vi "test - Response of CSM Send Message.vi"(8 "error in (no error)":errorcluster, 11 "TestCase in":refnum<class "testcase-Basic-Function.lvclass">) -> (0 "error out":errorcluster, 3 "TestCase out":refnum<class "testcase-Basic-Function.lvclass">)   [LabVIEW 2017, in "testcase-Basic-Function.lvclass"]
uses:
  testcase-Basic-Function.lvclass
  src/user.lib/_NEVSTOP/Communicable State Machine(CSM)/AdvanceAPI/CSM - Revert Arguments-Safe String.vi
  src/user.lib/_NEVSTOP/Communicable State Machine(CSM)/_Shared/Trim Single-line Text.vi
  src/user.lib/_NEVSTOP/Communicable State Machine(CSM)/AdvanceAPI/CSM - Make String Arguments Safe.vi
  src/user.lib/_NEVSTOP/Communicable State Machine(CSM)/AdvanceAPI/CSM - Break Down Multiple States String.vi
  src/user.lib/_NEVSTOP/Communicable State Machine(CSM)/AdvanceAPI/CSM - Compact Multiple States.vi
  src/user.lib/_NEVSTOP/Communicable State Machine(CSM)/AdvanceAPI/CSM - Keywords.vi
  src/user.lib/_NEVSTOP/Communicable State Machine(CSM)/Communicable State Machine.lvlib
  <vilib>/addons/_JKI Toolkits/VI Tester/TestCase.llb/TestCase.lvclass
  C:/Program Files (x86)/National Instruments/LabVIEW 2017/vi.lib/addons/_JKI Toolkits/VI Tester/TestCase.llb/TestCase.lvclass
panel:
  in  "response not empty in error handler":bool
  out "State History":string
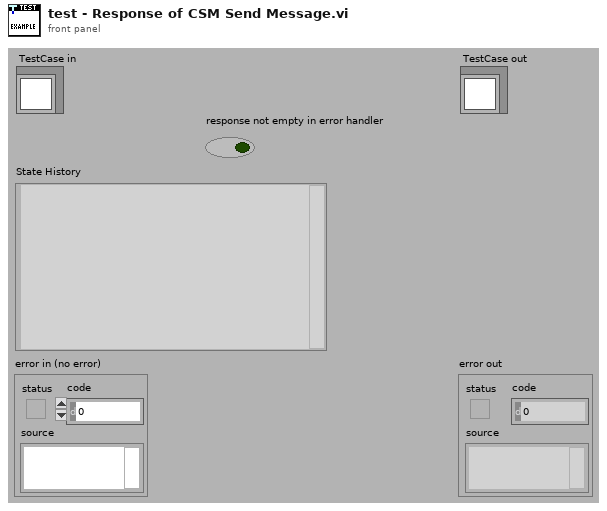
[diagram p1: front panel]
types:
  T1 = enum32{"Invalid", "Standard", "Closed", "Hidden", "Minimized", "Maximized"}
  T2 = enum32{"invalid app kind", "Development System", "Run Time System", "Student Edition", "Embedded LabVIEW", "Evaluation", "Custom"}
  T3 = typedef "Communicable State Machine.lvlib/_CSM_Response Source Message.ctl" = cluster{"‘State":string, "’Arguments":string, "’Error":errorcluster}
  T4 = cluster{"Current VI Reference":refnum<vi>, "Close Panel on Exit?":bool}
  T5 = cluster{"Core":cluster{"Current VI Reference":refnum<vi>, "Close Panel on Exit?":bool}, "Your Boolean data":bool, "Your string data":string}
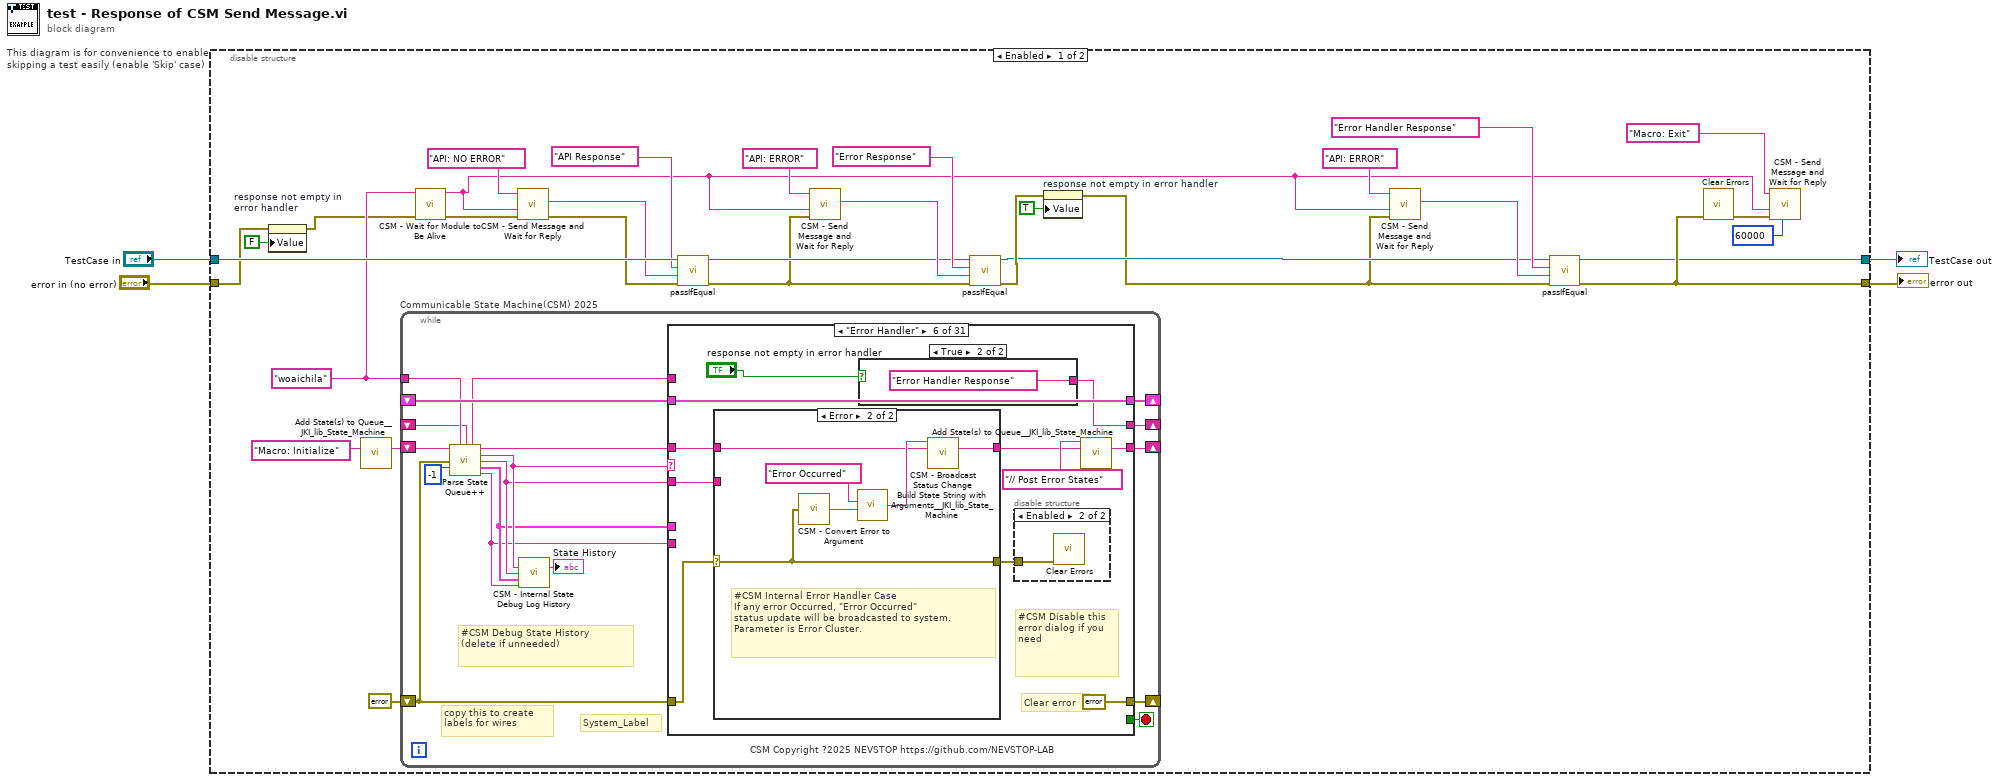
[diagram p0: block diagram]
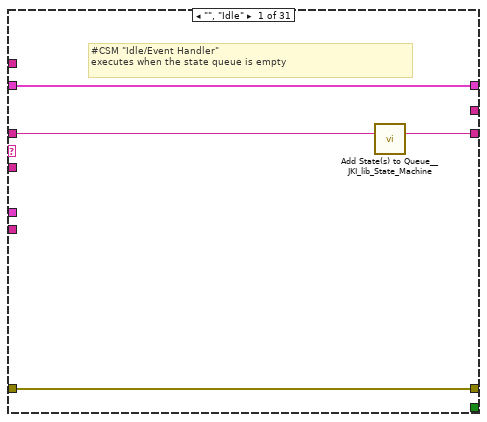
[diagram p2: hidden frame]
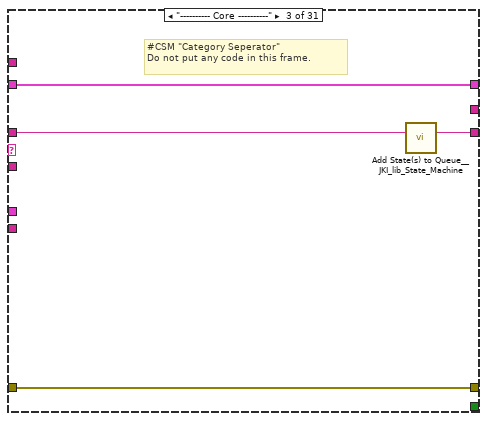
[diagram p4: hidden frame]
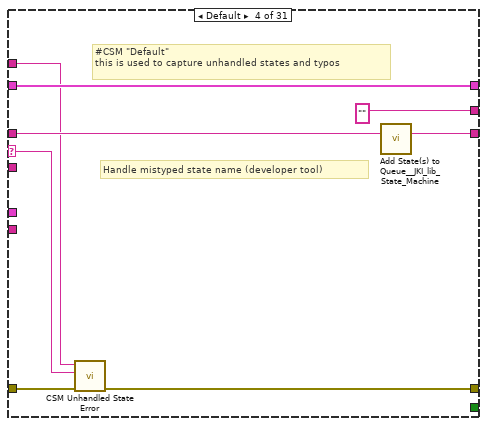
[diagram p5: hidden frame]
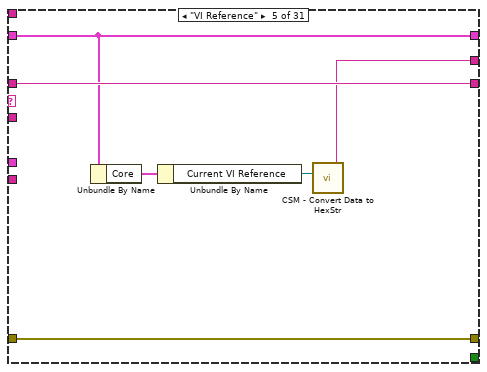
[diagram p6: hidden frame]
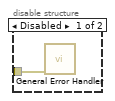
[diagram p8: hidden frame]
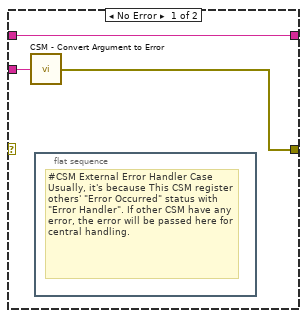
[diagram p9: hidden frame]
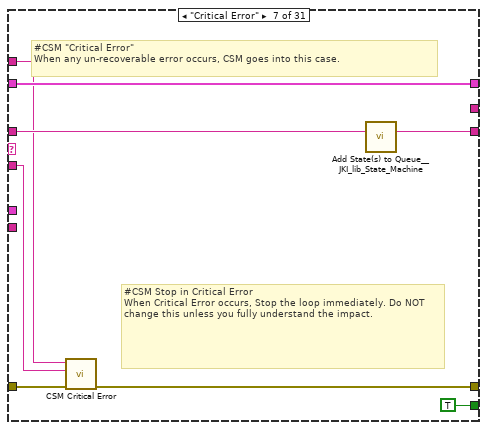
[diagram p10: hidden frame]
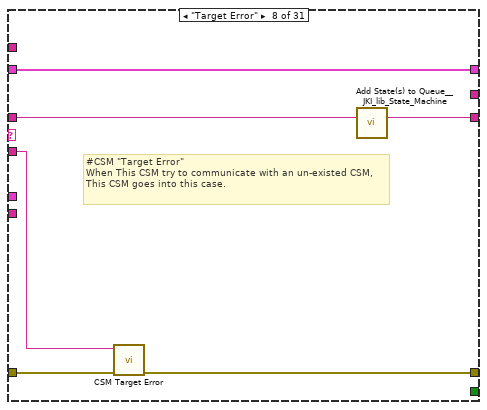
[diagram p11: hidden frame]
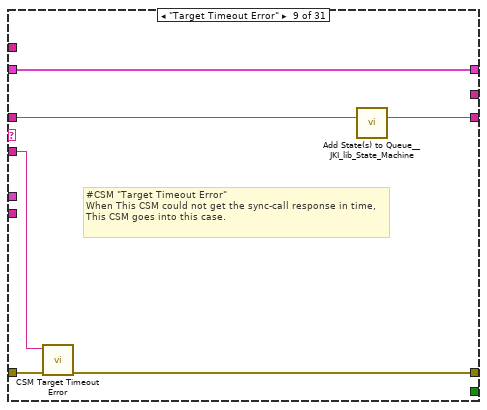
[diagram p12: hidden frame]
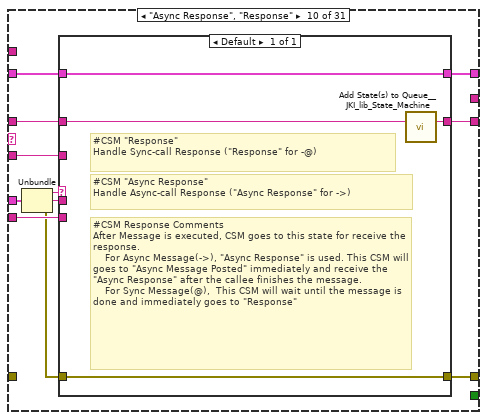
[diagram p13: hidden frame]
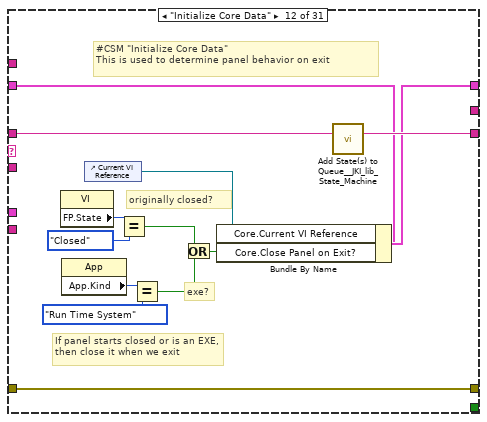
[diagram p15: hidden frame]
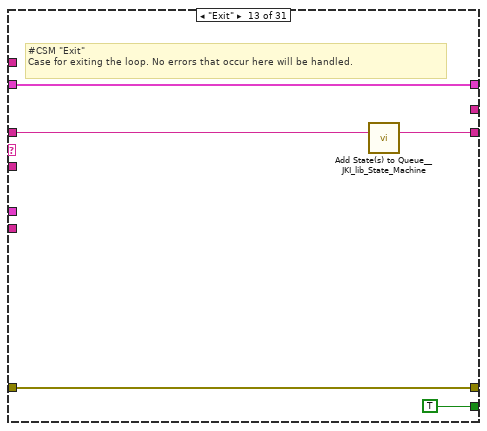
[diagram p16: hidden frame]
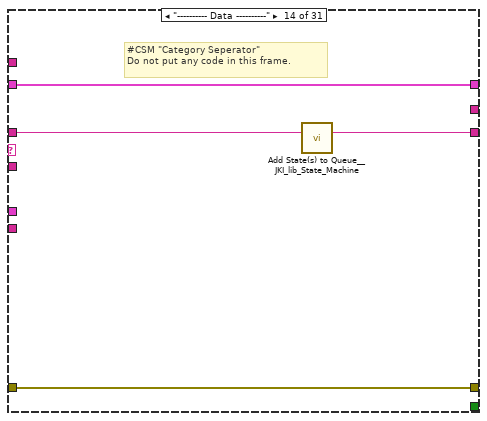
[diagram p17: hidden frame]
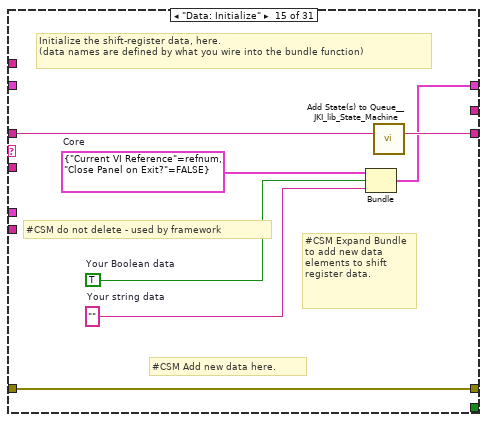
[diagram p18: hidden frame]
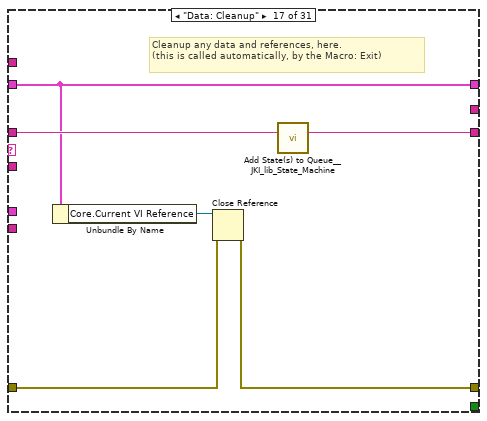
[diagram p20: hidden frame]
diagram:
  n1 = disable-structure "This diagram is for convenience to enable skipping a test easily (enable 'Skip' case)" shown="Enabled" {
    disable-tunnel: "TestCase in" -> [w35 w321]
    disable-tunnel: [w6 w319] -> w1
    disable-tunnel: [w8 w320] -> w3
    disable-tunnel: "error in (no error)" -> [w17 w318]
    frame Enabled {
      w30 = "woaichila" ("Name (\"\" to Use UUID)")
      n2 = property on="response not empty in error handler" class="Bool (strict)"(error in=w17, "Value"=FALSE ("response not empty in error handler")) -> (error out=w16:errorcluster)  [unwired: 1 in, 1 out]
      n3 = call <vilib>:"Add State(s) to Queue__JKI_lib_State_Machine.vi"("State(s) in (\"\")"="Macro: Initialize" ("Init State(\"Macro: Initialize\")")) -> ("States Out"=w32:string)  [unwired: 14 in]
      n4 = while "Communicable State Machine(CSM) 2025" {
        shift-right: [w48] -> _
        shift-left: _ -> [w47]
        shift-right: [w51] -> _
        shift-left: errorcluster {"status"=FALSE, "code"=0, "source"=""} ("error out") -> [w46]
        shift-right: [w50] -> _
        shift-left: w32 -> [w52]
        tunnel: w30 -> [w44]
        shift-right: [w45] -> _
        shift-left: _ -> [w38]
        stop <- w49 stop-if-true
        # "#CSM Debug State History\n(delete if unneeded)"
        # "copy this to create labels for wires"
        # "System_Label"
        # "CSM Copyright ?2025 NEVSTOP https://github.com/NEVSTOP-LAB"
        n5 = call "Parse State Queue++.vi"("State Queue"=w52, "Name (\"\" to Use UUID)"=w44, "Response Arguments"=w38, "Previous Error"=w46, "Dequeue (1 ms)"=-1 ("Timeout")) -> ("Name Used"=w39:string, "Remaining States"=w53:string, "Current State"=w43:string, "Arguments"=w42:string, "Additional Information"=w41:T3, "Source CSM"=w40:string)  [unwired: 5 in]
        n6 = call "CSM - Internal State Debug Log History.vi"("State"=w43, "Arguments (\"\")"=w42, ">> Response Source Message >>"=w41, "Source (\"\")"=w40) -> ("Debug Log"=→"State History":string)  [unwired: 11 in]
        n7 = case shown="\"Error Handler\"" w43 {
          selector: w43 -> [_ _ _ w67 _ _ _ _ _ _ _ _ _ _ _ _ _ _ _ _ _ _ _ _ _ _ _ _ _ _ _]
          tunnel: w53 -> [w54 w59 w64 w71 w77 w85 w107 w113 w119 w127 w138 w152 w157 w161 w168 w170 w177 w181 w185 w191 w206 w275 w280 w287 w289 w293 w298 w302 w309 w313 w317]
          tunnel: w42 -> [_ _ _ _ _ w84 w103 w112 w117 w126 _ _ _ _ _ _ _ _ _ w186 w200 _ _ _ _ _ _ w300 _ _ _]
          tunnel: w47 -> [w55 w58 w61 w69 w76 w88 w108 w114 w120 w129 w137 w145 w155 w158 _ w169 w172 w178 w183 w189 w202 w272 w277 w284 w288 w292 w297 w301 w306 w310 w314]
          tunnel: [w56 w60 w62 w65 w78 errorcluster {"status"=FALSE, "code"=0, "source"=""} ("error out") w104 w110 w116 w132 w139 w149 w154 w159 w165 w171 w173 w179 w182 w187 w203 w273 w278 w285 w290 w294 errorcluster {"status"=TRUE, "code"=-1, "source"="xxxx"} ("error out") w303 w307 w311 w315] -> w51
          tunnel: w46 -> [w56 w60 w62 w72 w78 w86 w109 w111 w118 _ w139 w149 w154 w159 w165 w171 w174 w179 w182 w188 w204 w273 w278 w285 w290 w294 _ w303 w307 w311 w315]
          tunnel: [w57 w59 w63 w70 w77 w81 w106 w115 w121 w128 w138 w151 w156 w160 w167 w170 w176 w180 w184 w190 w205 w274 w279 w286 w289 w293 w298 w302 w308 w312 w316] -> w50
          tunnel: [_ _ _ _ _ _ TRUE _ _ _ _ _ TRUE _ _ _ _ _ _ _ _ _ _ _ _ _ _ _ _ _ _] -> w49
          tunnel: [w55 w58 w61 w69 w76 w88 w108 w114 w120 w130 w137 w150 w155 w158 w166 w169 w172 w178 w183 w189 w202 w272 w277 w284 w288 w292 w297 w301 w306 w310 w314] -> w48
          tunnel: w40 -> [_ _ _ _ _ _ _ _ _ w124 _ _ _ _ _ _ _ _ _ _ _ _ _ _ _ _ _ _ _ _ _]
          tunnel: w41 -> [_ _ _ _ _ _ _ _ _ w131 _ _ _ _ _ _ _ _ _ _ _ _ _ _ _ _ _ _ _ _ _]
          tunnel: [_ _ _ "" w73 w80 _ _ _ _ _ _ _ _ _ _ _ _ _ _ _ _ _ _ _ "API Response" "Error Response" w299 _ _ _] -> w45
          tunnel: w39 -> [_ _ _ w66 _ _ w102 _ _ _ _ _ _ _ _ _ _ _ _ _ _ _ _ _ _ _ _ _ _ _ _]
          frame "", "Idle" {
            # "#CSM \"Idle/Event Handler\"\nexecutes when the state queue is empty"
            n8 = call <vilib>:"Add State(s) to Queue__JKI_lib_State_Machine.vi"("State(s) in (\"\")"=w54) -> ("States Out"=w57:string)  [unwired: 14 in]
          }
          frame "CSM Documentation" {
            # "#CSM README FIRST\n\nCommunicable State Machine(CSM) is a LabVIEW application framework that builds upon JKI State Machine(JKISM). It follows the pattern of JKISM and extends the keywords to describe message communication between modules, including concepts such as Sync-Message, Async-Message, Subscription/Unsubscription of status - essential elements for creating reusable code modules. For more information, please visit the CSM wiki: https://nevstop-lab.github.io/CSM-Wiki/\n\nFor instructions on JKI State Machine, visit: http://jki.net/state-machine/\nFor information about CSM, visit: https://github.com/NEVSTOP-LAB"
            # "#CSM \"Documentation\"\nCase for holding CSM Documenation"
          }
          frame "---------- Core ----------" {
            # "#CSM \"Category Seperator\"\nDo not put any code in this frame."
            n9 = call <vilib>:"Add State(s) to Queue__JKI_lib_State_Machine.vi"("State(s) in (\"\")"=w64) -> ("States Out"=w63:string)  [unwired: 14 in]
          }
          frame Default {
            # "#CSM \"Default\"\nthis is used to capture unhandled states and typos"
            # "Handle mistyped state name (developer tool)"
            n10 = call "CSM Unhandled State Error.vi"("error in (no error)"=w72, "Undefined State"=w67, "CSM Name"=w66) -> ("error out"=w65:errorcluster)  [unwired: 8 in]
            n11 = call <vilib>:"Add State(s) to Queue__JKI_lib_State_Machine.vi"("State(s) in (\"\")"=w71) -> ("States Out"=w70:string)  [unwired: 14 in]
          }
          frame "VI Reference" {
            n12 = Unbundle By Name(w76) -> ("Core"=w75:T4)
            n13 = Unbundle By Name(w75) -> ("Current VI Reference"=w74:refnum<vi>)
            n14 = call "CSM - Convert Data to HexStr.vi"("Variant"=w74) -> ("HEX String (0-9,A-F)"=w73:string)  [unwired: 8 in]
          }
          frame "Error Handler" {
            # "#CSM Disable this error dialog if you need"
            # "Clear error"
            n15 = case shown="Error" w86 {
              selector: w86 -> [_ w96]
              tunnel: [w95 w98] -> w82
              tunnel: w85 -> [w95 w97]
              tunnel: w84 -> [w94 _]
              tunnel: [w93 w96] -> w87
              frame No Error {
                n16 = call "CSM - Convert Argument to Error.vi"("Argument"=w94) -> ("Error"=w93:errorcluster)  [unwired: 4 in]
                n17 = flat-sequence {
                  frame #0 {
                    # "#CSM External Error Handler Case\nUsually, it's because This CSM register others' \"Error Occurred\" status with \"Error Handler\". If other CSM have any error, the error will be passed here for central handling."
                  }
                }
              }
              frame Error {
                # "#CSM Internal Error Handler Case \nIf any error Occurred, \"Error Occurred\" \nstatus update will be broadcasted to system.\nParameter is Error Cluster."
                n18 = call "CSM - Convert Error to Argument.vi"("Error"=w96) -> ("Argument"=w100:string)  [unwired: 4 in]
                n19 = call <vilib>:"Build State String with Arguments__JKI_lib_State_Machine.vi"("Arguments (\"\")"=w100, "State"="Error Occurred" ("Status with Arguments")) -> ("State with Arguments"=w99:string)  [unwired: 4 in]
                n20 = call "CSM - Broadcast Status Change.vi"("Status With Arguments"=w99, "State Queue"=w97) -> ("Remaining States"=w98:string)  [unwired: 13 in]
              }
            }
            n21 = case shown="True" "response not empty in error handler" {
              tunnel: [_ "Error Handler Response"] -> w80
              frame False {
              }
              frame True {
              }
            }
            n22 = disable-structure shown="Enabled" {
              disable-tunnel: w87 -> [w91 w92]
              frame Disabled {
                n23 = call <vilib>:"General Error Handler.vi"("error in (no error)"=w91) -> ()  [unwired: 10 in, 5 out]
              }
              frame Enabled {
                n24 = call <vilib>:"Clear Errors.vi"("error in (no error)"=w92) -> ()  [unwired: 5 in, 2 out]
              }
            }
            n25 = call <vilib>:"Add State(s) to Queue__JKI_lib_State_Machine.vi"("State(s) in Front (\"\")"="// Post Error States", "State(s) in (\"\")"=w82) -> ("States Out"=w81:string)  [unwired: 13 in]
          }
          frame "Critical Error" {
            # "#CSM Stop in Critical Error\nWhen Critical Error occurs, Stop the loop immediately. Do NOT change this unless you fully understand the impact."
            # "#CSM \"Critical Error\"\nWhen any un-recoverable error occurs, CSM goes into this case."
            n26 = call "CSM Critical Error.vi"("error in (no error)"=w109, "Arugments (As Reason)"=w103, "CSM Name"=w102) -> ("error out"=w104:errorcluster)  [unwired: 8 in]
            n27 = call <vilib>:"Add State(s) to Queue__JKI_lib_State_Machine.vi"("State(s) in (\"\")"=w107) -> ("States Out"=w106:string)  [unwired: 14 in]
          }
          frame "Target Error" {
            # "#CSM \"Target Error\"\nWhen This CSM try to communicate with an un-existed CSM, This CSM goes into this case."
            n28 = call "CSM Target Error.vi"("error in (no error)"=w111, "Arguments (As CSM Name)"=w112) -> ("error out"=w110:errorcluster)  [unwired: 9 in]
            n29 = call <vilib>:"Add State(s) to Queue__JKI_lib_State_Machine.vi"("State(s) in (\"\")"=w113) -> ("States Out"=w115:string)  [unwired: 14 in]
          }
          frame "Target Timeout Error" {
            # "#CSM \"Target Timeout Error\"\nWhen This CSM could not get the sync-call response in time, This CSM goes into this case."
            n30 = call "CSM Target Timeout Error.vi"("error in (no error)"=w118, "Arguments (As CSM Name)"=w117) -> ("error out"=w116:errorcluster)  [unwired: 9 in]
            n31 = call <vilib>:"Add State(s) to Queue__JKI_lib_State_Machine.vi"("State(s) in (\"\")"=w119) -> ("States Out"=w121:string)  [unwired: 14 in]
          }
          frame "Async Response", "Response" {
            n32 = Unbundle(w131) -> ("‘State"=w125:string, "’Arguments"=w123:string, "’Error"=w122:errorcluster)
            n33 = case shown="Default" w125 {
              tunnel: [w136] -> w132
              tunnel: w122 -> [w136]
              tunnel: [w135] -> w130
              tunnel: w129 -> [w135]
              tunnel: [w133] -> w128
              tunnel: w127 -> [w134]
              tunnel: w126 -> [_]
              tunnel: w124 -> [_]
              tunnel: w123 -> [_]
              frame Default {
                # "#CSM Response Comments\nAfter Message is executed, CSM goes to this state for receive the response.\n    For Async Message(->), \"Async Response\" is used. This CSM will goes to \"Async Message Posted\" immediately and receive the \"Async Response\" after the callee finishes the message.\n    For Sync Message(@),  This CSM will wait until the message is done and immediately goes to \"Response\""
                # "#CSM \"Async Response\"\nHandle Async-call Response (\"Async Response\" for ->)"
                # "#CSM \"Response\"\nHandle Sync-call Response (\"Response\" for -@)"
                n34 = call <vilib>:"Add State(s) to Queue__JKI_lib_State_Machine.vi"("State(s) in (\"\")"=w134) -> ("States Out"=w133:string)  [unwired: 14 in]
              }
            }
          }
          frame "Async Message Posted" {
            # "#CSM \"Async Message Posted\"\nAfter Async Message is posted (-> or ->| ), CSM goes to this state for post-action.\nYou can use Argument - State to tell which Async Message is called."
          }
          frame "Initialize Core Data" {
            # "#CSM \"Initialize Core Data\"\nThis is used to determine panel behavior on exit"
            # "originally closed?"
            # "exe?"
            # "If panel starts closed or is an EXE, then close it when we exit"
            n35 = property class="VI"() -> ("FP.State"=w142:T1)  [unwired: 2 in, 2 out]
            n36 = property class="App"() -> ("App.Kind"=w148:T2)  [unwired: 2 in, 2 out]
            n37 = control-ref of="Current VI Reference"() -> (w143:refnum<vi>)
            n38 = Equal?(x=w142, y=T1."Closed" ("Front Panel Window:State")) -> (x = y?=w140:bool)
            n39 = Equal?(x=w148, y=T2."Run Time System" ("Application:Kind")) -> (x = y?=w146:bool)
            n40 = Or(x=w140, y=w146) -> (x .or. y?=w144:bool)
            n41 = Bundle By Name(cluster=w145, "Core.Current VI Reference"=w143, "Core.Close Panel on Exit?"=w144) -> (w150:T5)
            n42 = call <vilib>:"Add State(s) to Queue__JKI_lib_State_Machine.vi"("State(s) in (\"\")"=w152) -> ("States Out"=w151:string)  [unwired: 14 in]
          }
          frame "Exit" {
            # "#CSM \"Exit\"\nCase for exiting the loop. No errors that occur here will be handled."
            n43 = call <vilib>:"Add State(s) to Queue__JKI_lib_State_Machine.vi"("State(s) in (\"\")"=w157) -> ("States Out"=w156:string)  [unwired: 14 in]
          }
          frame "---------- Data ----------" {
            # "#CSM \"Category Seperator\"\nDo not put any code in this frame."
            n44 = call <vilib>:"Add State(s) to Queue__JKI_lib_State_Machine.vi"("State(s) in (\"\")"=w161) -> ("States Out"=w160:string)  [unwired: 14 in]
          }
          frame "Data: Initialize" {
            w162 = T4 {"Current VI Reference"=refnum, "Close Panel on Exit?"=FALSE}  # Core
            w164 = TRUE  # Your Boolean data
            w163 = ""  # Your string data
            # "#CSM do not delete - used by framework"
            # "#CSM Expand Bundle to add new data elements to shift register data."
            # "#CSM Add new data here."
            # "Initialize the shift-register data, here.\n(data names are defined by what you wire into the bundle function)"
            n45 = Bundle("Core"=w162, "Your Boolean data"=w164, "Your string data"=w163) -> (w166:T5)  [unwired: 1 in]
            n46 = call <vilib>:"Add State(s) to Queue__JKI_lib_State_Machine.vi"("State(s) in (\"\")"=w168) -> ("States Out"=w167:string)  [unwired: 14 in]
          }
          frame "Data: Update Indicators" {
          }
          frame "Data: Cleanup" {
            # "Cleanup any data and references, here.\n(this is called automatically, by the Macro: Exit)"
            n47 = Unbundle By Name(w172) -> ("Core.Current VI Reference"=w175:refnum<vi>)
            n48 = Close Reference(reference=w175, error in (no error)=w174) -> (error out=w173:errorcluster)
            n49 = call <vilib>:"Add State(s) to Queue__JKI_lib_State_Machine.vi"("State(s) in (\"\")"=w177) -> ("States Out"=w176:string)  [unwired: 14 in]
          }
          frame "---------- UI ----------" {
            # "#CSM \"Category Seperator\"\nDo not put any code in this frame."
            n50 = call <vilib>:"Add State(s) to Queue__JKI_lib_State_Machine.vi"("State(s) in (\"\")"=w181) -> ("States Out"=w180:string)  [unwired: 14 in]
          }
          frame "UI: Initialize" {
            # "#CSM \"UI: Initialize\"\nInitialize the User Interface, here.\n(this is called automatically, by the Macro: Init)"
            n51 = call <vilib>:"Add State(s) to Queue__JKI_lib_State_Machine.vi"("State(s) in (\"\")"=w185) -> ("States Out"=w184:string)  [unwired: 14 in]
          }
          frame "UI: Cursor Set" {
            # "#CSM \"UI: Cursor Set\"\nSet and Unset Cursor Busy.\n(Usage: \"UI: Cursor Set >> Busy|Idle\")"
            # "Argument"
            n52 = disable-structure shown="TARGET_TYPE!=Windows" {
              disable-tunnel: w188 -> [w194 w199]
              disable-tunnel: [w193 w199] -> w187
              disable-tunnel: w186 -> [w192 _]
              frame condition #0 (active) {
                n53 = case shown="\"Idle\", Default" w192 {
                  tunnel: w194 -> [w196 w198]
                  tunnel: [w195 w197] -> w193
                  frame "Idle", Default {
                    n54 = call <vilib>:"Unset Busy.vi"("error in (no error)"=w196) -> ("error out"=w195:errorcluster)  [unwired: 10 in]
                  }
                  frame "Busy" {
                    n55 = call <vilib>:"Set Busy.vi"("error in (no error)"=w198) -> ("error out"=w197:errorcluster)  [unwired: 9 in, 1 out]
                  }
                }
              }
              frame condition #1 {
              }
            }
            n56 = call <vilib>:"Add State(s) to Queue__JKI_lib_State_Machine.vi"("State(s) in (\"\")"=w191) -> ("States Out"=w190:string)  [unwired: 14 in]
          }
          frame "UI: Front Panel State" {
            # "#CSM \"UI: Front Panel State\"\nSet Front Panel Open or Closed\n(Usage: \"UI: Front Panel State >> Open|Close\")"
            # "Argument"
            n57 = Unbundle By Name(w202) -> ("Core.Current VI Reference"=w201:refnum<vi>)
            n58 = call <vilib>:"Add State(s) to Queue__JKI_lib_State_Machine.vi"("State(s) in (\"\")"=w206) -> ("States Out"=w205:string)  [unwired: 14 in]
            n59 = case shown="\"Close\", \"Closed\"" w200 {
              tunnel: w204 -> [w212 w227 w238 w251 w264]
              tunnel: [w214 w228 w240 w253 w266] -> w203
              tunnel: w201 -> [w213 w225 w239 w252 w265]
              frame "Open", "Standard", Default {
                w207 = T1."Standard" ("State")
                n60 = property class="VI"(reference=w213, error in=w212) -> (reference out=w210:refnum<vi>, error out=w211:errorcluster, "FP.State"=w209:T1)
                n61 = Not Equal?(x=w209, y=w207) -> (x != y?=w208:bool)
                n62 = case shown="True" w208 {
                  tunnel: [w218 w220] -> w214
                  tunnel: w211 -> [w217 w220]
                  tunnel: w210 -> [w216 _]
                  tunnel: w207 -> [w215 _]
                  frame True {
                    n63 = invoke class="VI" method="FP.Open"(reference=w216, error in=w217, "Activate"=TRUE, "State"=w215) -> (error out=w218:errorcluster)  [unwired: 1 in, 4 out]
                  }
                  frame False {
                  }
                }
              }
              frame "Close", "Closed" {
                n64 = property class="VI"(reference=w225, error in=w227) -> (reference out=w224:refnum<vi>, error out=w226:errorcluster, "FP.State"=w222:T1)
                n65 = Not Equal?(x=w222, y=T1."Closed" ("Front Panel Window:State")) -> (x != y?=w221:bool)
                n66 = case shown="False" w221 {
                  tunnel: [w229 w232] -> w228
                  tunnel: w226 -> [w229 w231]
                  tunnel: w224 -> [_ w230]
                  frame False {
                  }
                  frame True {
                    n67 = invoke class="VI" method="FP.Close"(reference=w230, error in=w231) -> (error out=w232:errorcluster)  [unwired: 1 in, 2 out]
                  }
                }
              }
              frame "Hidden", "Hide" {
                w233 = T1."Hidden" ("State")
                n68 = property class="VI"(reference=w239, error in=w238) -> (reference out=w236:refnum<vi>, error out=w237:errorcluster, "FP.State"=w235:T1)
                n69 = Not Equal?(x=w235, y=w233) -> (x != y?=w234:bool)
                n70 = case shown="True" w234 {
                  tunnel: [w244 w245] -> w240
                  tunnel: w237 -> [w243 w245]
                  tunnel: w236 -> [w242 _]
                  tunnel: w233 -> [w241 _]
                  frame True {
                    n71 = invoke class="VI" method="FP.Open"(reference=w242, error in=w243, "State"=w241) -> (error out=w244:errorcluster)  [unwired: 2 in, 4 out]
                  }
                  frame False {
                  }
                }
              }
              frame "Minimize", "Minimized" {
                w246 = T1."Minimized" ("State")
                n72 = property class="VI"(reference=w252, error in=w251) -> (reference out=w249:refnum<vi>, error out=w250:errorcluster, "FP.State"=w248:T1)
                n73 = Not Equal?(x=w248, y=w246) -> (x != y?=w247:bool)
                n74 = case shown="True" w247 {
                  tunnel: [w257 w258] -> w253
                  tunnel: w250 -> [w256 w258]
                  tunnel: w249 -> [w255 _]
                  tunnel: w246 -> [w254 _]
                  frame True {
                    n75 = invoke class="VI" method="FP.Open"(reference=w255, error in=w256, "State"=w254) -> (error out=w257:errorcluster)  [unwired: 2 in, 4 out]
                  }
                  frame False {
                  }
                }
              }
              frame "Maximize", "Maximized" {
                w259 = T1."Maximized" ("State")
                n76 = property class="VI"(reference=w265, error in=w264) -> (reference out=w262:refnum<vi>, error out=w263:errorcluster, "FP.State"=w261:T1)
                n77 = Not Equal?(x=w261, y=w259) -> (x != y?=w260:bool)
                n78 = case shown="True" w260 {
                  tunnel: [w270 w271] -> w266
                  tunnel: w263 -> [w269 w271]
                  tunnel: w262 -> [w268 _]
                  tunnel: w259 -> [w267 _]
                  frame True {
                    n79 = invoke class="VI" method="FP.Open"(reference=w268, error in=w269, "State"=w267) -> (error out=w270:errorcluster)  [unwired: 2 in, 4 out]
                  }
                  frame False {
                  }
                }
              }
            }
          }
          frame "---------- Macro ----------" {
            # "#CSM \"Category Seperator\"\nDo not put any code in this frame."
            n80 = call <vilib>:"Add State(s) to Queue__JKI_lib_State_Machine.vi"("State(s) in (\"\")"=w275) -> ("States Out"=w274:string)  [unwired: 14 in]
          }
          frame "Macro: Initialize" {
            # "#CSM \"Macro: Initialize\"\nInitialization Macro (This is called once, when the VI starts)"
            n81 = call <vilib>:"Add State(s) to Queue__JKI_lib_State_Machine.vi"("State(s) in Front (\"\")"="Data: Initialize\nInitialize Core Data\nData: Update Indicators", "State(s) in (\"\")"=w280) -> ("States Out"=w279:string)  [unwired: 13 in]
          }
          frame "Macro: Exit" {
            # "#CSM \"Macro: Exit\"\nExit Macro (This is called once, when the VI exits)"
            n82 = call <vilib>:"Add State(s) to Queue__JKI_lib_State_Machine.vi"("State(s) in Front (\"\")"="//Exit Sub-Modules ", "State(s) at Back (\"\")"="Data: Cleanup\nExit") -> ("States Out"=w282:string)  [unwired: 13 in]
            n83 = call <vilib>:"Add State(s) to Queue__JKI_lib_State_Machine.vi"("State(s) in Front (\"\")"=w282, "State(s) in (\"\")"=w287) -> ("States Out"=w286:string)  [unwired: 13 in]
          }
          frame "---------- API ----------" {
            # "#CSM \"Category Seperator\"\nDo not put any code in this frame."
          }
          frame "API: NO ERROR" {
            # "#CSM API Example\nCopy/Rename this case for your own API"
          }
          frame "API: ERROR" {
          }
          frame "API: API2" {
            # "#CSM API Example\nCopy/Rename this case for your own API"
            # "unpack Hex String  to Variant\nif complex parameter is needed."
            n84 = call "CSM - Convert HexStr to Data.vi"("HEX String"=w300) -> ()  [unwired: 7 in, 2 out]
            n85 = disable-structure shown="Disabled" {
              disable-tunnel: [w304 "API2 Response"] -> w299
              frame Disabled {
                # "pack variant to hexstr \nif complex response is needed."
                # "complex Response"
                n86 = call "CSM - Convert Data to HexStr.vi"() -> ("HEX String (0-9,A-F)"=w304:string)  [unwired: 9 in]
              }
              frame Enabled {
              }
            }
          }
          frame "---------- Action ----------" {
            # "#CSM \"Category Seperator\"\nDo not put any code in this frame."
            n87 = call <vilib>:"Add State(s) to Queue__JKI_lib_State_Machine.vi"("State(s) in (\"\")"=w309) -> ("States Out"=w308:string)  [unwired: 14 in]
          }
          frame "Action: action1" {
            # "#CSM \"Internal State\"\nThis category is used for holding internal states"
            n88 = call <vilib>:"Add State(s) to Queue__JKI_lib_State_Machine.vi"("State(s) in (\"\")"=w313) -> ("States Out"=w312:string)  [unwired: 14 in]
          }
          frame "Action: action2" {
            # "#CSM \"Internal State\"\nThis category is used for holding internal states"
            n89 = call <vilib>:"Add State(s) to Queue__JKI_lib_State_Machine.vi"("State(s) in (\"\")"=w317) -> ("States Out"=w316:string)  [unwired: 14 in]
          }
        }
      }
      n90 = call "CSM - Wait for Module to Be Alive.vi"("CSM Name"=w30, "error in (no error)"=w16) -> ("CSM Name (Dup)"=w7:string, "error out"=w31:errorcluster)  [unwired: 11 in, 1 out]
      n91 = call "CSM - Send Message and Wait for Reply.vi"("Error In (No Error)"=w31, "Target Module"=w7, "State"="API: NO ERROR" ("Name (\"\" to Use UUID)")) -> ("error out"=w29:errorcluster, "Response"=w27:string)  [unwired: 6 in, 1 out]
      n92 = call-dynamic "passIfEqual.vi"("error in (no error)"=w29, "y"=w27, "x"="API Response", "TestCase in"=w35) -> ("error out"=w19:errorcluster, "TestCase out"=w20:refnum<class "testcase-Basic-Function.lvclass">)  [unwired: 6 in]
      n93 = call "CSM - Send Message and Wait for Reply.vi"("Error In (No Error)"=w19, "Target Module"=w7, "State"="API: ERROR" ("Name (\"\" to Use UUID)")) -> ("Response"=w22:string)  [unwired: 6 in, 2 out]
      n94 = call-dynamic "passIfEqual.vi"("error in (no error)"=w19, "y"=w22, "x"="Error Response", "TestCase in"=w20) -> ("error out"=w14:errorcluster, "TestCase out"=w10:refnum<class "testcase-Basic-Function.lvclass">)  [unwired: 6 in]
      n95 = property on="response not empty in error handler" class="Bool (strict)"(error in=w14, "Value"=TRUE ("response not empty in error handler")) -> (error out=w9:errorcluster)  [unwired: 1 in, 1 out]
      n96 = call "CSM - Send Message and Wait for Reply.vi"("Error In (No Error)"=w9, "Target Module"=w7, "State"="API: ERROR" ("Name (\"\" to Use UUID)")) -> ("Response"=w12:string)  [unwired: 6 in, 2 out]
      n97 = call-dynamic "passIfEqual.vi"("error in (no error)"=w9, "y"=w12, "x"="Error Handler Response", "TestCase in"=w10) -> ("error out"=w8:errorcluster, "TestCase out"=w6:refnum<class "testcase-Basic-Function.lvclass">)  [unwired: 6 in]
      n98 = call <vilib>:"Clear Errors.vi"("error in (no error)"=w8) -> ("error out"=w25:errorcluster)  [unwired: 5 in, 1 out]
      n99 = call "CSM - Send Message and Wait for Reply.vi"("Response Timeout (-2 Using Global Settings)"=60000, "Error In (No Error)"=w25, "Target Module"=w7, "State"="Macro: Exit" ("Name (\"\" to Use UUID)")) -> ()  [unwired: 5 in, 3 out]
    }
    frame Disabled {
      # "skip test result while test is under development"
      n100 = call <vilib>:"skip.vi"("error in (no error)"=w318, "TestCase in"=w321) -> ("error out"=w320:errorcluster, "TestCase out"=w319:refnum<class "testcase-Basic-Function.lvclass">)  [unwired: 8 in]
    }
  }
  "error out" <- w3
  "TestCase out" <- w1
